vi "Init SPI.vi"(8 "error in (no error)":errorcluster, 9 "Name":string, 10 "DMA FIFO ref in":refnum<k20>, 11 "Device Ref in":T1 format="%.0x") -> (0 "error out":errorcluster, 1 "Compiled Info":T2 {"UEGO Engine Data"."Ordered Channels" format="%.0x"; "UEGO Engine Data"."RT IDs"."Slot #" max=15; "UEGO Engine Data"."RT IDs"."Chip Address (A2 A1 A0)" max=7; "DIO Engine Data"."Ordered Channels" format="%.0x"; "DIO Engine Data"."RT IDs"."Slot #" max=15; "DIO Engine Data"."RT IDs"."Chip Address (A2 A1 A0)" max=7; "LED Engine Data"."Ordered Channels" format="%.0x"; "LED Engine Data"."RT IDs"."Slot #" max=15; "LED Engine Data"."RT IDs"."Chip Address (A2 A1 A0)" max=7; "Current Sense Engine Data"."Ordered Channels" format="%.0x"; "Current Sense Engine Data"."RT IDs"."Slot #" max=15; "Current Sense Engine Data"."RT IDs"."Chip Address (A2 A1 A0)" max=7; "Resistor Engine Data"."Ordered Channels" format="%.0x"; "Resistor Engine Data"."RT IDs"."Slot #" max=15; "Resistor Engine Data"."RT IDs"."Chip Address (A2 A1 A0)" max=7; "Wheel Speed Sensor Engine Data"."Ordered Channels" format="%.0x"; "Wheel Speed Sensor Engine Data"."RT IDs"."Slot #" max=15; "Wheel Speed Sensor Engine Data"."RT IDs"."Chip Address (A2 A1 A0)" max=7; "Battery Switch Engine Data"."Ordered Channels" format="%.0x"; "Battery Switch Engine Data"."RT IDs"."Slot #" max=15; "Battery Switch Engine Data"."RT IDs"."Chip Address (A2 A1 A0)" max=7; "FIU Engine Data"."Ordered Channels" format="%.0x"; "FIU Engine Data"."RT IDs"."Slot #" max=15; "FIU Engine Data"."RT IDs"."Chip Address (A2 A1 A0)" max=7}, 3 "Device Ref out":T1 format="%.0x")   [LabVIEW 2014, in "SLSC configuration Engine.lvlib"]
uses:
  SLSC configuration Engine.lvlib
  <vilib>/NI Veristand/Custom Device API/Custom Device Item Ref.ctl
  Shared/Type Defs/SLSC compiled.ctl
  Shared/Type Defs/RT Engine Data.ctl
  Shared/Type Defs/RT IDs.ctl
  Shared/SPI Utility/Slot #.ctl
  Shared/MCP23S17/Chip Address.ctl
  Type Defs/RT UEGO Setting Time Data.ctl
  Shared/SLSC configuration Shared.lvlib
  <vilib>/NI Veristand/Custom Device API/Custom Device API.lvlib
  System Explorer/SLSC configuration System Explorer.lvlib
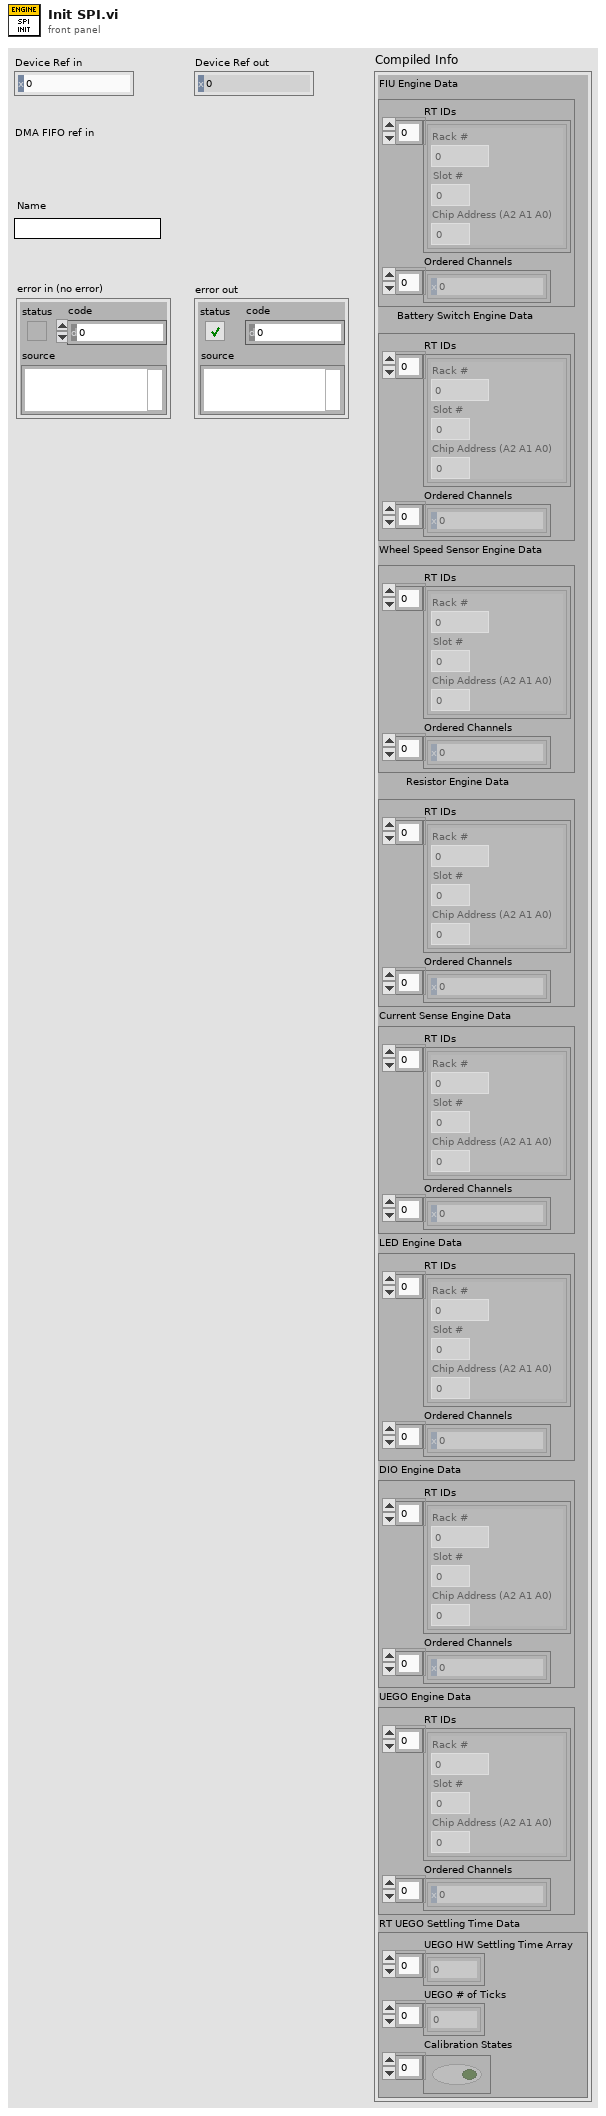
[diagram p1: front panel]
types:
  T1 = typedef "Custom Device API.lvlib/Custom Device Item Ref.ctl" = u64
  T2 = typedef "SLSC configuration Shared.lvlib/SLSC compiled.ctl" = cluster{"FIU Engine Data":T3, "Battery Switch Engine Data":T3, "Wheel Speed Sensor Engine Data":T3, "Resistor Engine Data":T3, "Current Sense Engine Data":T3, "LED Engine Data":T3, "DIO Engine Data":T3, "UEGO Engine Data":T3, "RT UEGO Settling Time Data":T7}
  T3 = typedef "SLSC configuration Shared.lvlib/RT Engine Data.ctl" = cluster{"RT IDs":T4[], "Ordered Channels":T1[]}
  T4 = typedef "SLSC configuration Shared.lvlib/RT IDs.ctl" = cluster{"Rack #":u8, "Slot #":T5, "Chip Address (A2 A1 A0)":T6}
  T5 = typedef "SLSC configuration Shared.lvlib/Slot #.ctl" = u8
  T6 = typedef "SLSC configuration Shared.lvlib/Chip Address.ctl" = u8
  T7 = typedef "SLSC configuration Engine.lvlib/RT UEGO Setting Time Data.ctl" = cluster{"UEGO HW Settling Time Array":u32[], "UEGO # of Ticks":u32[], "Calibration States":bool[]}
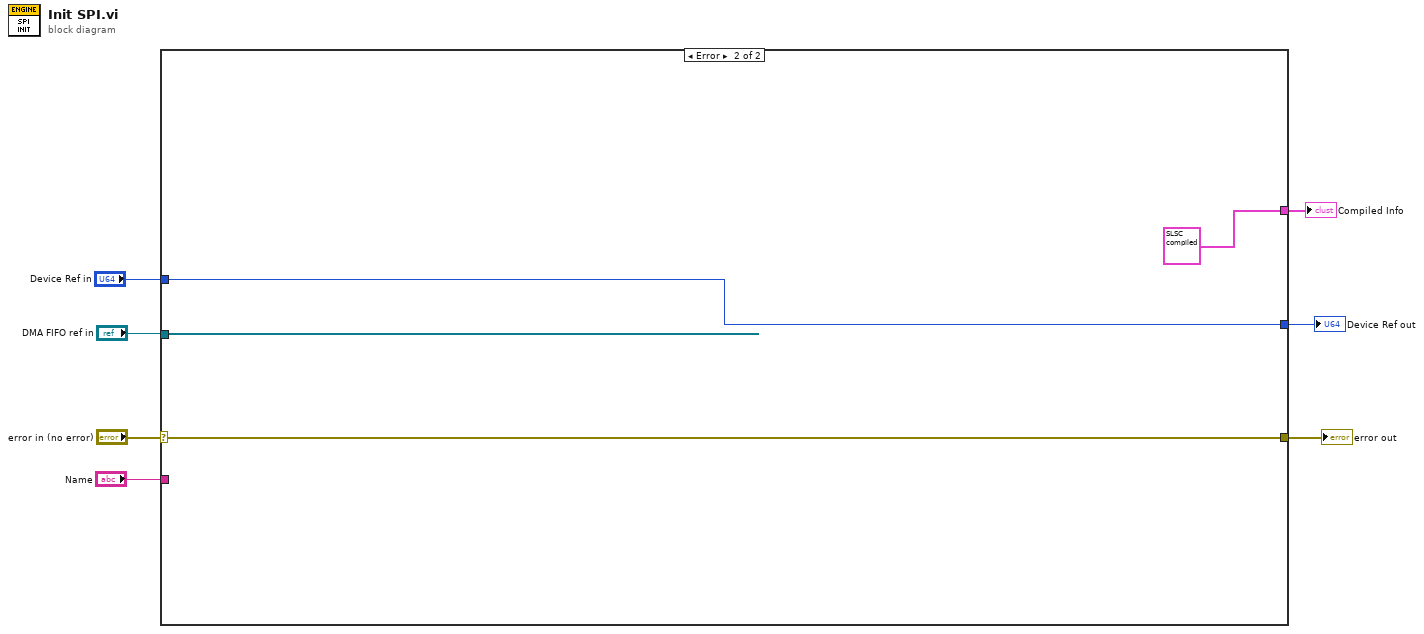
[diagram p0: block diagram]
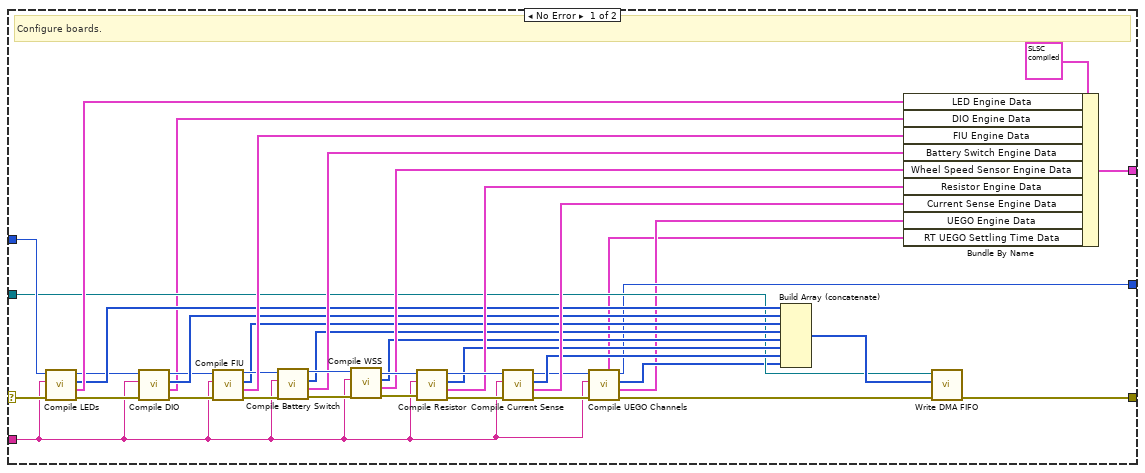
[diagram p2: hidden frame]
diagram:
  n1 = case shown="Error" "error in (no error)" {
    selector: "error in (no error)" -> [w21 w51]
    tunnel: "DMA FIFO ref in" -> [w17 _]
    tunnel: [w18 w51] -> w7
    tunnel: "Device Ref in" -> [w20 w49]
    tunnel: [w26 T2 {"FIU Engine Data"={"RT IDs"=[], "Ordered Channels"=[]}, "Battery Switch Engine Data"={"RT IDs"=[], "Ordered Channels"=[]}, "Wheel Speed Sensor Engine Data"={"RT IDs"=[], "Ordered Channels"=[]}, "Resistor Engine Data"={"RT IDs"=[], "Ordered Channels"=[]}, "Current Sense Engine Data"={"RT IDs"=[], "Ordered Channels"=[]}, "LED Engine Data"={"RT IDs"=[], "Ordered Channels"=[]}, "DIO Engine Data"={"RT IDs"=[], "Ordered Channels"=[]}, "UEGO Engine Data"={"RT IDs"=[], "Ordered Channels"=[]}, "RT UEGO Settling Time Data"={"UEGO HW Settling Time Array"=[], "UEGO # of Ticks"=[], "Calibration States"=[]}} ("type")] -> w4
    tunnel: [w13 w49] -> w2
    tunnel: "Name" -> [w9 _]
    frame No Error {
      # "Configure boards."
      n2 = call "Compile LEDs.vi"("error in (no error)"=w21, "Name"=w9, "Device Item Ref in"=w20) -> ("error out"=w23:errorcluster, "LEDs Engine Data"=w25:T3, "Initial LEDs SPI CMDs"=w24:u64[], "Device Item Ref out"=w22:T1)  [unwired: 5 in]
      n3 = call "Compile DIO.vi"("error in (no error)"=w23, "Name"=w9, "Device Item Ref in"=w22) -> ("error out"=w27:errorcluster, "DIO Engine Data"=w16:T3, "Initial DIO SPI CMDs"=w30:u64[], "Device Item Ref out"=w28:T1)  [unwired: 5 in]
      n4 = call "Compile FIU.vi"("error in (no error)"=w27, "Name"=w9, "Device Item Ref in"=w28) -> ("error out"=w32:errorcluster, "FIU Engine Data"=w48:T3, "Initial FIU SPI CMDs"=w31:u64[], "Device Item Ref out"=w33:T1)  [unwired: 5 in]
      n5 = call "Compile Battery Switch.vi"("error in (no error)"=w32, "Name"=w9, "Device Item Ref in"=w33) -> ("error out"=w36:errorcluster, "Battery Switch Engine Data"=w35:T3, "Initial Battery Switch SPI CMDs"=w34:u64[], "Device Item Ref out"=w37:T1)  [unwired: 5 in]
      n6 = call "Compile WSS.vi"("error in (no error)"=w36, "Name"=w9, "Device Item Ref in"=w37) -> ("error out"=w40:errorcluster, "Wheel Speed Sensor Engine Data"=w39:T3, "Initial Wheel Speed Sensor SPI CMDs"=w38:u64[], "Device Item Ref out"=w41:T1)  [unwired: 5 in]
      n7 = call "Compile Resistor.vi"("error in (no error)"=w40, "Name"=w9, "Device Item Ref in"=w41) -> ("error out"=w44:errorcluster, "Resistor Engine Data"=w43:T3, "Initial Resistor SPI CMDs"=w42:u64[], "Device Item Ref out"=w45:T1)  [unwired: 5 in]
      n8 = call "Compile Current Sense.vi"("error in (no error)"=w44, "Name"=w9, "Device Item Ref in"=w45) -> ("error out"=w15:errorcluster, "Wheel Speed Sensor Engine Data"=w47:T3, "Initial Wheel Speed Sensor SPI CMDs"=w46:u64[], "Device Item Ref out"=w14:T1)  [unwired: 5 in]
      n9 = call "Compile UEGO Channels.vi"("error in (no error)"=w15, "Name"=w9, "Device Item Ref in"=w14) -> ("error out"=w12:errorcluster, "UEGO Engine Data"=w10:T3, "Initial UEGO SPI CMDs"=w11:u64[], "Device Item Ref out"=w13:T1, "RT UEGO Settling Time Data"=w8:T7)  [unwired: 4 in]
      n10 = Build Array (concatenate)(w24, w30, w31, w34, w38, w42, w46, w11) -> (w19:u64[])
      n11 = Bundle By Name(cluster=T2 {"FIU Engine Data"={"RT IDs"=[], "Ordered Channels"=[]}, "Battery Switch Engine Data"={"RT IDs"=[], "Ordered Channels"=[]}, "Wheel Speed Sensor Engine Data"={"RT IDs"=[], "Ordered Channels"=[]}, "Resistor Engine Data"={"RT IDs"=[], "Ordered Channels"=[]}, "Current Sense Engine Data"={"RT IDs"=[], "Ordered Channels"=[]}, "LED Engine Data"={"RT IDs"=[], "Ordered Channels"=[]}, "DIO Engine Data"={"RT IDs"=[], "Ordered Channels"=[]}, "UEGO Engine Data"={"RT IDs"=[], "Ordered Channels"=[]}, "RT UEGO Settling Time Data"={"UEGO HW Settling Time Array"=[], "UEGO # of Ticks"=[], "Calibration States"=[]}} ("SLSC Compiled out"), "LED Engine Data"=w25, "DIO Engine Data"=w16, "FIU Engine Data"=w48, "Battery Switch Engine Data"=w35, "Wheel Speed Sensor Engine Data"=w39, "Resistor Engine Data"=w43, "Current Sense Engine Data"=w47, "UEGO Engine Data"=w10, "RT UEGO Settling Time Data"=w8) -> (w26:T2)
      n12 = call "Write DMA FIFO.vi"("error in (no error)"=w12, "FIU SPI Commands"=w19, "DMA FIFO Ref in"=w17) -> ("error out"=w18:errorcluster)  [unwired: 8 in]
    }
    frame Error {
    }
  }
  "error out" <- w7
  "Compiled Info" <- w4
  "Device Ref out" <- w2
